vi "Test2.vi"() -> ()   [LabVIEW 2013]
uses:
  <vilib>/Motion/MotorControl/_s/nism.interpretControlRegister.stateTransition.ctl
  <vilib>/rvi/Emulation/niFpgaSctlEmulationGetInTimedLoop.vi
  <vilib>/rvi/Emulation/niFpgaEmulationReportErrorSimple.vi
  <vilib>/rvi/Emulation/niFpgaGetClockAttributes.vi
  Global FPGA.vi
  <vilib>/Motion/MotorControl/_s/nism.interpretControlRegister.indexed.vi
  <vilib>/Motion/MotorControl/_s/nism.generateStatusRegister.indexed.vi
  <vilib>/rvi/Emulation/niFpgaProcessEmulError.vi
  <vilib>/Motion/MotorControl/_s/nism.mdo.read.dio.portA.2.vi
  <vilib>/Motion/MotorControl/_s/nism.mdo.read.positionLoopSyncData.vi
  <vilib>/Motion/MotorControl/_s/nism.mdo.read.splineData.vi
  <vilib>/rvi/eio/common/nirviEmuTemplateMethod_errors.vi
  <vilib>/rvi/Emulation/niFpgaCriticalErrorInLSC.vi
  <vilib>/eio/EIONode/EIONode.xnode
  <vilib>/Motion/MotorControl/NI_SoftMotion_MotorControlIP.lvlib
panel:
  out "State":T1=enum."Start --> Initializing" caption="state transition"
  in  "Drive Enable override?":bool
  in  "Enable value":bool
  out "Drive Enable":bool[](array[boolean])
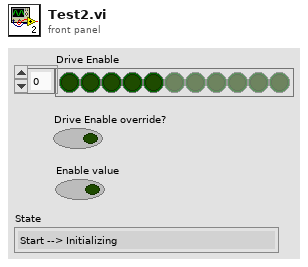
[diagram p1: front panel]
types:
  T1 = typedef "NI_SoftMotion_MotorControlIP.lvlib/nism.interpretControlRegister.stateTransition.ctl" = enum8{"Invalid", "Start --> Initializing", "Initializing --> Disabled", "Disabled --> Ready To Switch On", "Ready To Switch On --> Switched On", "Ready To Switch On --> Disable", "Switched On --> Operation Enable", "Switched On --> Ready To Switch On", "Switched On --> Disabled", "Operation Enable --> Switched On", "Operation Enable --> Ready To Switch On", "Operation Enable --> Disabled", "Fault --> Disabled", "Any --> Fault", "None"}
  T2 = typedef "NI_SoftMotion_MotorControlIP.lvlib/nism.dio.portA.config.2.ctl" = cluster{"digital filter (us)":u16[], "safe state":enum16{"Low", "High", "No Change"}[]}
  T3 = typedef "NI_SoftMotion_MotorControlIP.lvlib/nism.mdo.splineData.ctl" = cluster{"spline type":T4, "traj per/spline per":u16, "spline per/traj per":fxp<+,32,0>}
  T4 = typedef "nism.splineInterpolation.type.ctl" = u16
  T5 = typedef "NI_SoftMotion_Synchronization.lvlib/nism.softmotionScan.timerConfig.ctl" = cluster{"Target Period (clocks)":u16, "Host Period / Target Period":u16}
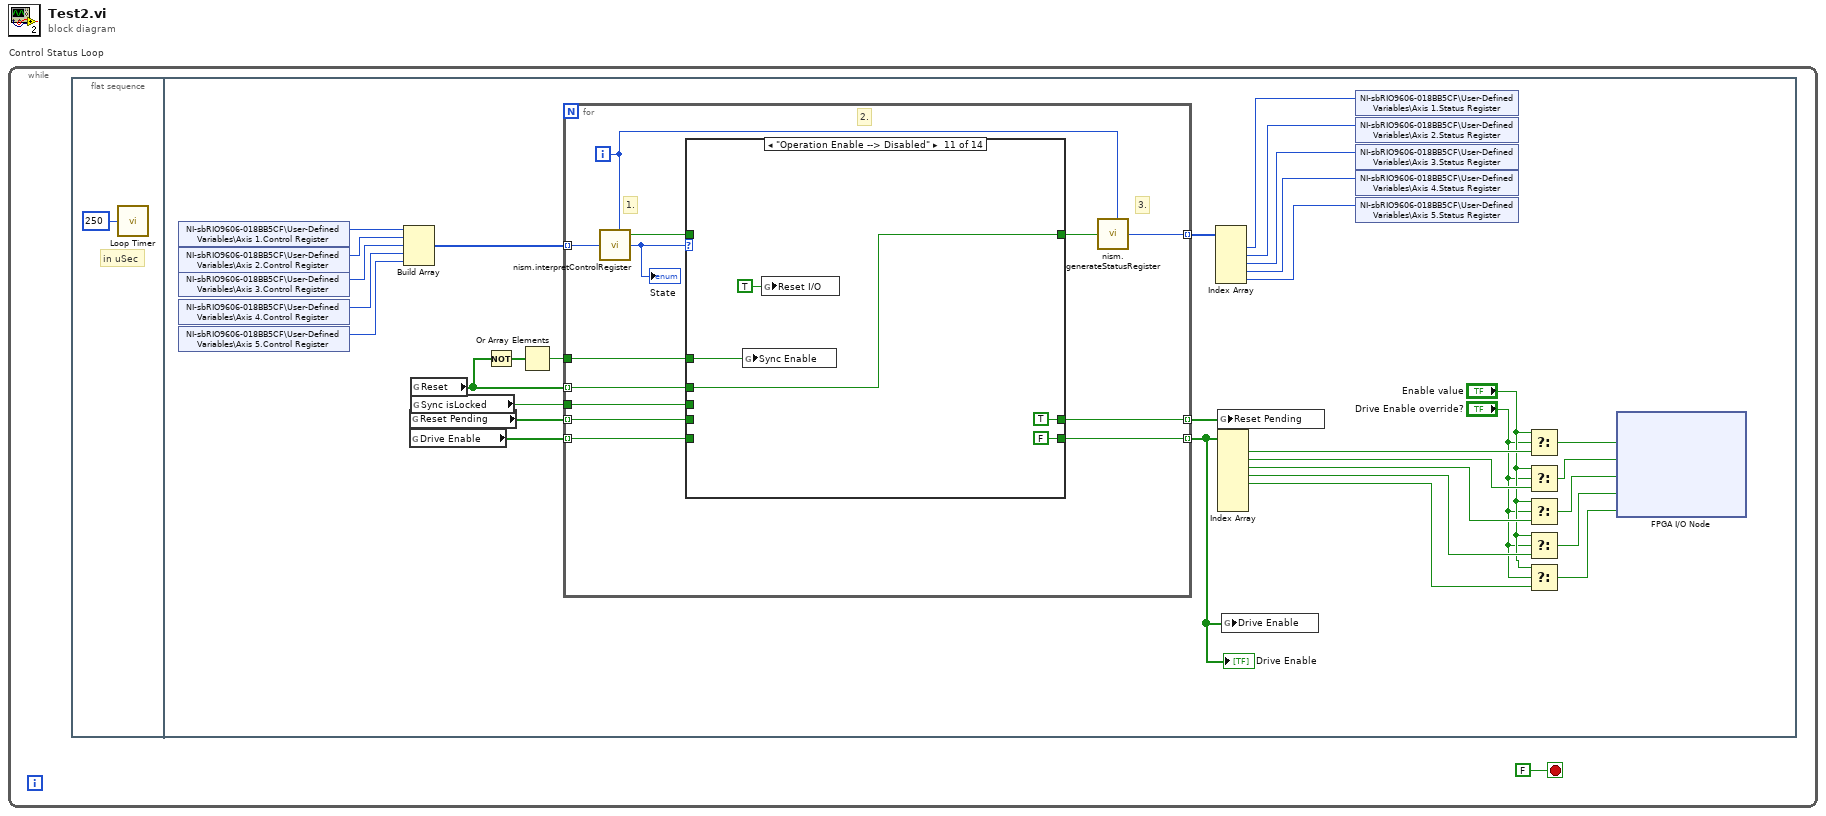
[diagram p0: block diagram]
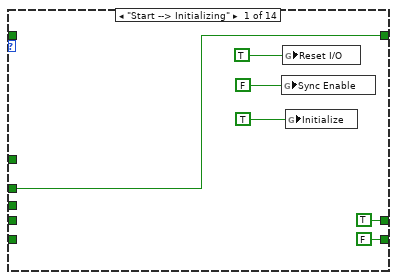
[diagram p2: hidden frame]
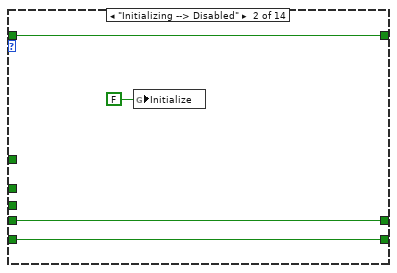
[diagram p3: hidden frame]
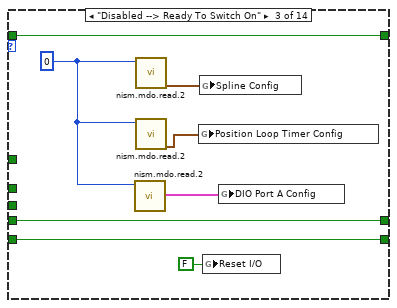
[diagram p4: hidden frame]
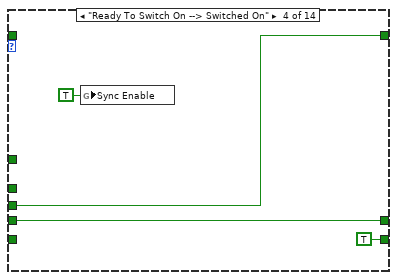
[diagram p5: hidden frame]
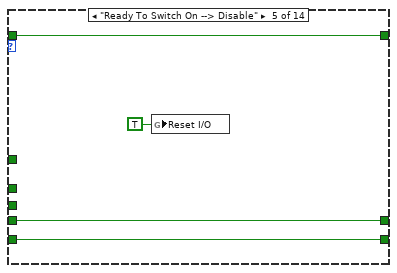
[diagram p6: hidden frame]
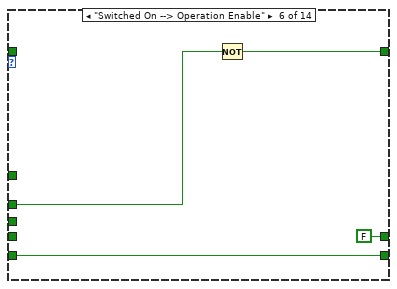
[diagram p7: hidden frame]
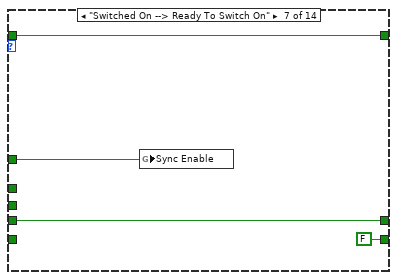
[diagram p8: hidden frame]
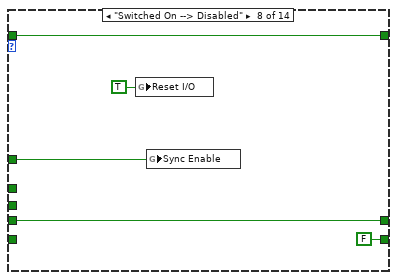
[diagram p9: hidden frame]
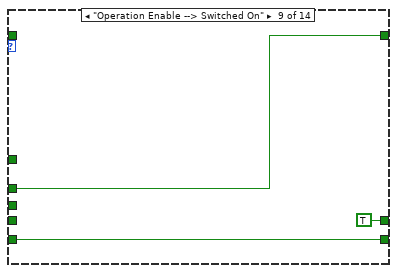
[diagram p10: hidden frame]
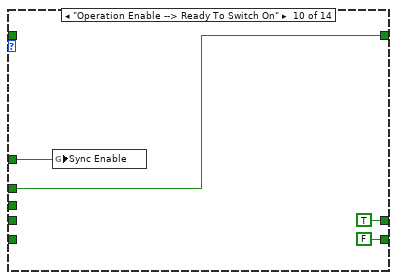
[diagram p11: hidden frame]
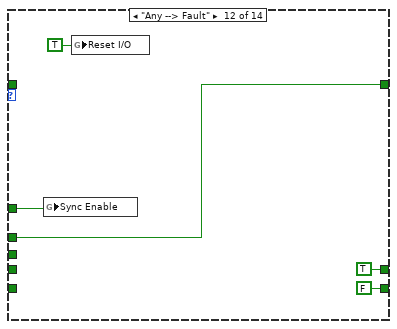
[diagram p12: hidden frame]
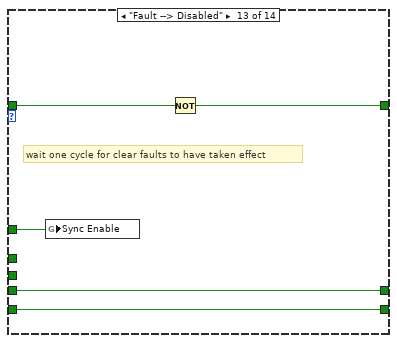
[diagram p13: hidden frame]
diagram:
  n1 = while "Control Status Loop" {
    stop <- FALSE stop-if-true
    n2 = flat-sequence {
      frame #0 {
        # "in uSec"
        n3 = call "Loop Timer"("Count(uSec)"=u32 250) -> ()  [unwired: 1 out]
      }
      frame #1 {
        n4 = shared-variable "NI-sbRIO9606-018BB5CF\\User-Defined Variables\\Axis 1.Control Register"() -> (w24:u32)  [unwired: 1 in, 1 out]
        n5 = shared-variable "NI-sbRIO9606-018BB5CF\\User-Defined Variables\\Axis 2.Control Register"() -> (w23:u32)  [unwired: 1 in, 1 out]
        n6 = shared-variable "NI-sbRIO9606-018BB5CF\\User-Defined Variables\\Axis 3.Control Register"() -> (w22:u32)  [unwired: 1 in, 1 out]
        n7 = shared-variable "NI-sbRIO9606-018BB5CF\\User-Defined Variables\\Axis 4.Control Register"() -> (w21:u32)  [unwired: 1 in, 1 out]
        n8 = shared-variable "NI-sbRIO9606-018BB5CF\\User-Defined Variables\\Axis 5.Control Register"() -> (w20:u32)  [unwired: 1 in, 1 out]
        n9 = Build Array(w24, w23, w22, w21, w20) -> (w33:u32[])
        n10 = global read "Global FPGA.vi" "Reset Pending"() -> (w28:bool[])
        n11 = global read "Global FPGA.vi" "Drive Enable"() -> (w27:bool[])
        n12 = global read "Global FPGA.vi" "Reset"() -> (w29:bool[])
        n13 = global read "Global FPGA.vi" "Sync isLocked"() -> (w34:bool)
        n14 = Not(x=w29) -> (.not. x?=w31:bool[])
        n15 = Or Array Elements(Boolean array=w31) -> (logical OR=w30:bool)
        n16 = for {
          tunnel: w29 -> [w42] mode=indexing
          tunnel: w34 -> [w41]
          tunnel: w33 -> [w43] mode=indexing
          tunnel: [w40] -> w25 mode=indexing
          tunnel: [w39] -> w32 mode=indexing
          tunnel: [w38] -> w26 mode=indexing
          tunnel: w30 -> [w37]
          tunnel: w28 -> [w36] mode=indexing
          tunnel: w27 -> [w35] mode=indexing
          i -> [w44]
          # "3."
          # "2."
          # "1."
          n17 = call-poly <vilib>:"nism.interpretControlRegister.vi"("control register"=w43, "axis index"=w44) -> ("transition occurred"=w45:bool, "state transition"=w46:T1)  [unwired: 6 in]
          "State" <- w46
          n18 = case shown="\"Operation Enable --> Disabled\"" w46 {
            tunnel: w45 -> [_ w57 w65 _ w73 _ w81 w86 _ _ _ _ w108 _]
            tunnel: [w53 w57 w65 w67 w73 w77 w81 w86 w88 w91 w96 w101 w107 _] -> w47
            tunnel: w42 -> [w53 _ _ _ _ w76 _ _ w88 w91 w96 w101 _ _]
            tunnel: w41 -> [_ _ _ w67 _ _ _ _ _ _ _ _ _ _]
            tunnel: [TRUE ("Write.Reset Pending") w56 w62 w66 w72 FALSE ("Write.Reset Pending") w78 w83 TRUE ("Write.Reset Pending") TRUE ("Write.Reset Pending") TRUE ("Write.Reset Pending") TRUE ("Write.Reset Pending") w105 w110] -> w39
            tunnel: [FALSE ("Write.Drive Enable") w55 w61 TRUE ("Write.Drive Enable") w71 w74 FALSE ("Write.Drive Enable") FALSE ("Write.Drive Enable") w87 FALSE ("Write.Drive Enable") FALSE ("Write.Drive Enable") FALSE ("Write.Drive Enable") w104 w109] -> w38
            tunnel: w37 -> [_ _ _ _ _ _ w79 w84 _ w90 w95 w100 w106 _]
            tunnel: w36 -> [_ w56 w62 w66 w72 _ w78 w83 _ _ _ _ w105 w110]
            tunnel: w35 -> [_ w55 w61 _ w71 w74 _ _ w87 _ _ _ w104 w109]
            frame "Start --> Initializing" {
              n19 = global write "Global FPGA.vi" "Sync Enable"(FALSE ("Sync Enable")) -> ()
              n20 = global write "Global FPGA.vi" "Reset I/O"(TRUE ("Reset I/O")) -> ()
              n21 = global write "Global FPGA.vi" "Initialize"(TRUE ("Reset I/O")) -> ()
            }
            frame "Initializing --> Disabled" {
              n22 = global write "Global FPGA.vi" "Initialize"(FALSE ("Reset I/O")) -> ()
            }
            frame "Disabled --> Ready To Switch On" {
              w59 = 0 ("axis index")
              n23 = call-poly <vilib>:"nism.mdo.read.2.vi"("axis index"=w59) -> ("dio config (port a)"=w58:T2)  [unwired: 10 in]
              n24 = call-poly <vilib>:"nism.mdo.read.2.vi"("axis index"=w59) -> ("spline"=w64:T3)  [unwired: 10 in]
              n25 = call-poly <vilib>:"nism.mdo.read.2.vi"("axis index"=w59) -> ("position loop sync"=w63:T5)  [unwired: 10 in]
              n26 = global write "Global FPGA.vi" "Position Loop Timer Config"(w63) -> ()
              n27 = global write "Global FPGA.vi" "Spline Config"(w64) -> ()
              n28 = global write "Global FPGA.vi" "Reset I/O"(FALSE ("Reset I/O")) -> ()
              n29 = global write "Global FPGA.vi" "DIO Port A Config"(w58) -> ()
            }
            frame "Ready To Switch On --> Switched On" {
              n30 = global write "Global FPGA.vi" "Sync Enable"(TRUE ("Sync Enable")) -> ()
            }
            frame "Ready To Switch On --> Disable" {
              n31 = global write "Global FPGA.vi" "Reset I/O"(TRUE ("Reset I/O")) -> ()
            }
            frame "Switched On --> Operation Enable" {
              n32 = Not(x=w76) -> (.not. x?=w77:bool)
            }
            frame "Switched On --> Ready To Switch On" {
              n33 = global write "Global FPGA.vi" "Sync Enable"(w79) -> ()
            }
            frame "Switched On --> Disabled" {
              n34 = global write "Global FPGA.vi" "Reset I/O"(TRUE ("Reset I/O")) -> ()
              n35 = global write "Global FPGA.vi" "Sync Enable"(w84) -> ()
            }
            frame "Operation Enable --> Switched On" {
            }
            frame "Operation Enable --> Ready To Switch On" {
              n36 = global write "Global FPGA.vi" "Sync Enable"(w90) -> ()
            }
            frame "Operation Enable --> Disabled" {
              n37 = global write "Global FPGA.vi" "Sync Enable"(w95) -> ()
              n38 = global write "Global FPGA.vi" "Reset I/O"(TRUE ("Reset I/O")) -> ()
            }
            frame "Any --> Fault" {
              n39 = global write "Global FPGA.vi" "Sync Enable"(w100) -> ()
              n40 = global write "Global FPGA.vi" "Reset I/O"(TRUE ("Reset I/O")) -> ()
            }
            frame "Fault --> Disabled" {
              # "wait one cycle for clear faults to have taken effect"
              n41 = global write "Global FPGA.vi" "Sync Enable"(w106) -> ()
              n42 = Not(x=w108) -> (.not. x?=w107:bool)
            }
            frame "None", Default {
            }
          }
          n43 = call-poly <vilib>:"nism.generateStatusRegister.vi"("transition success"=w47, "axis index"=w44) -> ("status register"=w40:u32)  [unwired: 7 in]
        }
        "Drive Enable" <- w26
        n44 = Index Array(array=w25) -> (element #1=w19:u32, element #2=w18:u32, element #3=w17:u32, element #4=w16:u32, element #5=w15:u32)  [unwired: 5 in]
        n45 = global write "Global FPGA.vi" "Reset Pending"(w32) -> ()
        n46 = Index Array(array=w26) -> (element #1=w14:bool, element #2=w12:bool, element #3=w10:bool, element #4=w8:bool, element #5=w6:bool)  [unwired: 8 in, 3 out]
        n47 = global write "Global FPGA.vi" "Drive Enable"(w26) -> ()
        n48 = shared-variable "NI-sbRIO9606-018BB5CF\\User-Defined Variables\\Axis 1.Status Register"(w19) -> ()  [unwired: 1 in, 1 out]
        n49 = shared-variable "NI-sbRIO9606-018BB5CF\\User-Defined Variables\\Axis 2.Status Register"(w18) -> ()  [unwired: 1 in, 1 out]
        n50 = shared-variable "NI-sbRIO9606-018BB5CF\\User-Defined Variables\\Axis 3.Status Register"(w17) -> ()  [unwired: 1 in, 1 out]
        n51 = shared-variable "NI-sbRIO9606-018BB5CF\\User-Defined Variables\\Axis 4.Status Register"(w16) -> ()  [unwired: 1 in, 1 out]
        n52 = shared-variable "NI-sbRIO9606-018BB5CF\\User-Defined Variables\\Axis 5.Status Register"(w15) -> ()  [unwired: 1 in, 1 out]
        n53 = Select(t="Enable value", s="Drive Enable override?", f=w14) -> (s? t:f=w13:bool)
        n54 = Select(t="Enable value", s="Drive Enable override?", f=w12) -> (s? t:f=w11:bool)
        n55 = Select(t="Enable value", s="Drive Enable override?", f=w10) -> (s? t:f=w9:bool)
        n56 = Select(t="Enable value", s="Drive Enable override?", f=w8) -> (s? t:f=w7:bool)
        n57 = Select(t="Enable value", s="Drive Enable override?", f=w6) -> (s? t:f=w5:bool)
        n58 = xnode "FPGA I/O Node"("Axis1_Servo On"=w13, "Axis2_Servo On"=w11, "Axis3_Servo On"=w9, "Axis4_Servo On"=w7, "Axis5_Servo On"=w5) -> ()  [unwired: 5 in, 5 out]
      }
    }
  }
